vi "VI-Wait For State.vi"(0 "VI ref":refnum<vi>, 9 "Timeout (s)":dbl=5.0, 11 "error in (no error)":errorcluster) -> (15 "error out":errorcluster)   [LabVIEW 2020]
uses:
  b612412e-8aec-4c51-bfe4-144552ef5e58.vi
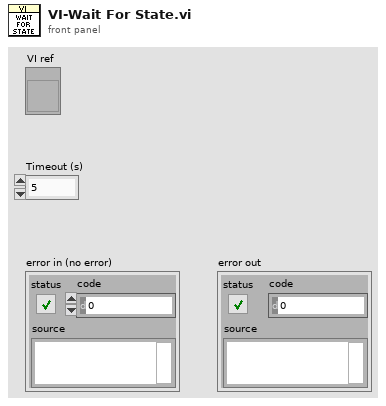
[diagram p1: front panel]
types:
  T1 = enum32{"Bad", "Idle", "Run top level", "Running"}
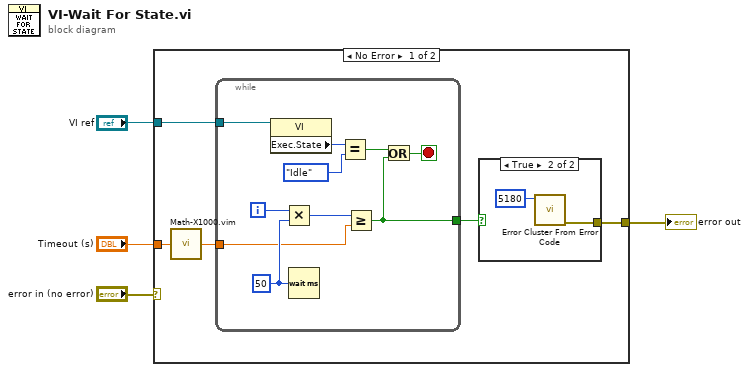
[diagram p0: block diagram]
diagram:
  n1 = case shown="No Error" "error in (no error)" {
    selector: "error in (no error)" -> [_ w22]
    tunnel: "VI ref" -> [w9 _]
    tunnel: "Timeout (s)" -> [w8 _]
    tunnel: [w5 w22] -> w2
    frame No Error {
      n2 = call "Math-X1000.vim"("X"=w8) -> ("1000X"=w7:dbl)
      n3 = while {
        tunnel: w9 -> [w19]
        tunnel: w7 -> [w14]
        tunnel: [w12] -> w6
        i -> [w17]
        stop <- w13 stop-if-true
        w18 = u32 50 ("milliseconds to wait")
        n4 = property class="VI"(reference=w19) -> ("Exec.State"=w21:T1)  [unwired: 1 in, 2 out]
        n5 = Multiply(x=w17, y=w18) -> (x*y=w15:u32)
        n6 = Wait (ms)(milliseconds to wait=w18) -> ()  [unwired: 1 out]
        n7 = Equal?(x=w21, y=T1."Idle" ("Execution:State")) -> (x = y?=w16:bool)
        n8 = Greater Or Equal?(x=w15, y=w14) -> (x >= y?=w12:bool)
        n9 = Or(x=w16, y=w12) -> (x .or. y?=w13:bool)
      }
      n10 = case shown="True" w6 {
        tunnel: [_ w11] -> w5
        frame False {
        }
        frame True {
          n11 = call <vilib>:"Error Cluster From Error Code.vi"("error code (0)"=5180) -> ("error out"=w11:errorcluster)  [unwired: 8 in]
        }
      }
    }
    frame Error {
    }
  }
  "error out" <- w2
